vi "UpdatingCurrentFolder.vi"(8 "에러 입력(에러 없음)":errorcluster, 11 ".NET 참조 번호 입력":refnum<k24>) -> (0 "에러 출력":errorcluster, 2 "ParsingName":string, 3 ".NET 참조 번호 출력":refnum<k24>)   [LabVIEW 2017, in "Retrieved Data.lvclass"]
uses:
  Retrieved Data.lvclass
  C:/Users/KimYG/Application/Solution Package/Minhee Retriever/binaries/Microsoft.WindowsAPICodePack.Shell.dll
  binaries/Microsoft.WindowsAPICodePack.Shell.dll
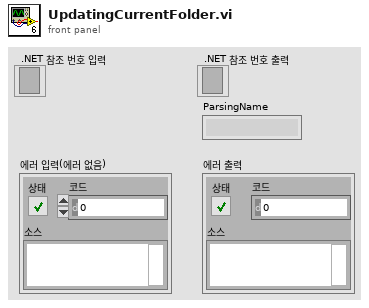
[diagram p1: front panel]
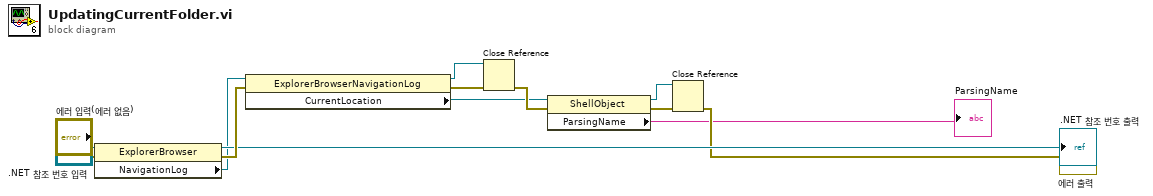
[diagram p0: block diagram]
diagram:
  n1 = property class="ExplorerBrowser"(reference=".NET 참조 번호 입력", error in="에러 입력(에러 없음)") -> (reference out=→".NET 참조 번호 출력":refnum<k24>, error out=w12:errorcluster, "NavigationLog"=w2:refnum<k24>)
  n2 = property class="ExplorerBrowserNavigationLog"(reference=w2, error in=w12) -> (reference out=w5:refnum<k24>, error out=w6:errorcluster, "CurrentLocation"=w1:refnum<k24>)
  n3 = Close Reference(reference=w5, error in (no error)=w6) -> (error out=w7:errorcluster)
  n4 = property class="ShellObject"(reference=w1, error in=w7) -> (reference out=w9:refnum<k24>, error out=w8:errorcluster, "ParsingName"=→"ParsingName":string)
  n5 = Close Reference(reference=w9, error in (no error)=w8) -> (error out=→"에러 출력":errorcluster)
